vi "testPLCm.vi"() -> ()   [LabVIEW 2011]
uses:
  <vilib>/Instr/_visa.llb/VISA Configure Serial Port (Instr).vi
panel:
  in  "停止":bool
  out "Y20-Y37":T1
  out "Y0-Y17":T2
  in  "停止位":u16(ring)=10 items=["1.0"=10, "1.5"=15, "2.0"=20]
  in  "校验位":enum16{"None", "Odd", "Even", "Mark", "Space"}(ring)=enum."Even"
  in  "数据位":u16=7
  in  "波特率":u32=9600
  in  "串口号":refnum<visa-resource-name>="COM3"
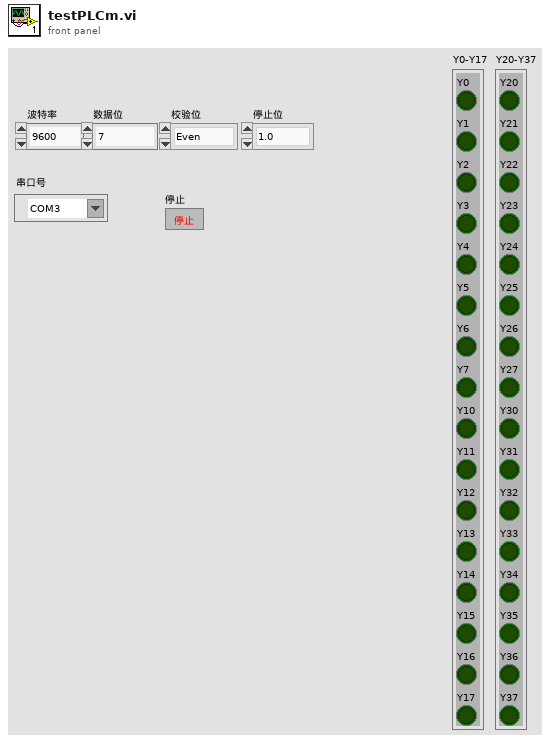
[diagram p1: front panel]
types:
  T1 = cluster{"Y20":bool, "Y21":bool, "Y22":bool, "Y23":bool, "Y24":bool, "Y25":bool, "Y26":bool, "Y27":bool, "Y30":bool, "Y31":bool, "Y32":bool, "Y33":bool, "Y34":bool, "Y35":bool, "Y36":bool, "Y37":bool}
  T2 = cluster{"Y0":bool, "Y1":bool, "Y2":bool, "Y3":bool, "Y4":bool, "Y5":bool, "Y6":bool, "Y7":bool, "Y10":bool, "Y11":bool, "Y12":bool, "Y13":bool, "Y14":bool, "Y15":bool, "Y16":bool, "Y17":bool}
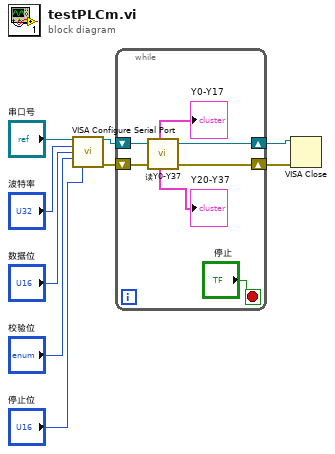
[diagram p0: block diagram]
diagram:
  n1 = call-poly "VISA Configure Serial Port"("VISA resource name"="串口号", "baud rate (9600)"="波特率", "data bits (8)"="数据位", "parity (0:none)"="校验位", "stop bits (10: 1 bit)"="停止位") -> ("VISA resource name out"=w4:refnum<visa-resource-name>, "error out"=w3:errorcluster)  [unwired: 9 in]
  n2 = while {
    shift-right: [w12] -> w2
    shift-left: w4 -> [w16]
    shift-right: [w11] -> w1
    shift-left: w3 -> [w15]
    stop <- "停止" stop-if-true
    n3 = call "读Y0-Y37.vi"("VISA资源名称"=w16, "错误输入（无错误）"=w15) -> ("Y0-Y17"=→"Y0-Y17":T2, "Y20-Y37"=→"Y20-Y37":T1, "VISA资源名称输出"=w12:refnum<visa-resource-name>, "错误输出"=w11:errorcluster)  [unwired: 4 in]
  }
  n4 = VISA Close(VISA resource name=w2, error in (no error)=w1) -> ()  [unwired: 1 out]
